vi "ABCtoDQ_noSine_2PhasePowerInvariant_src.vi"(0 "A":sgl, 1 "cosx":sgl, 2 "sinx":sgl, 5 "B":sgl) -> (4 "direct":sgl, 6 "quadrature":sgl, 10 "alpha":sgl, 15 "beta":sgl)   [LabVIEW 2017]
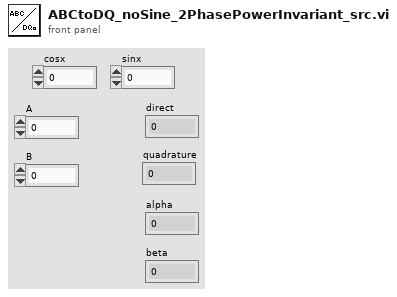
[diagram p1: front panel]
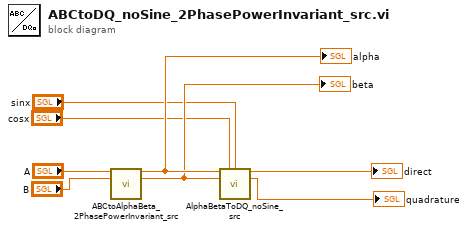
[diagram p0: block diagram]
diagram:
  n1 = call "ABCtoAlphaBeta_2PhasePowerInvariant_src.vi"("A"="A", "B"="B") -> ("alpha"=w4:sgl, "beta"=w3:sgl)  [unwired: 12 in]
  "alpha" <- w4
  "beta" <- w3
  n2 = call "AlphaBetaToDQ_noSine_src.vi"("alpha"=w4, "cosx"="cosx", "sinx"="sinx", "beta"=w3) -> ("direct"=→"direct":sgl, "quadrature"=→"quadrature":sgl)  [unwired: 10 in]
